vi "一体站流程自动启动.vi"(11 "参数":T1) -> ()   [LabVIEW 2016, in "PLC.lvlib"]
uses:
  PLC.lvlib
panel:
  out "s? t:f":enum16{"初始化", "采配水启动", "仪器操作", "反冲洗", "结束"}(ring)
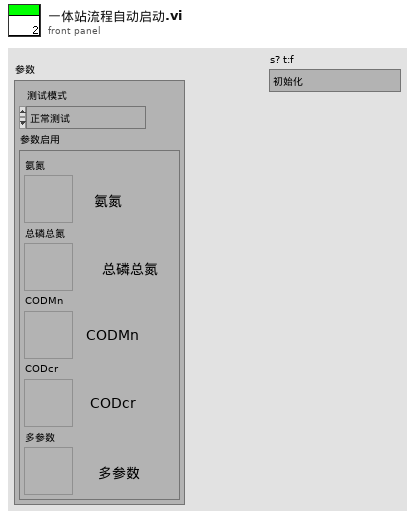
[diagram p1: front panel]
types:
  T1 = cluster{"测试模式":enum16{"正常测试", "集成干预"}, "参数启用":cluster{"氨氮":bool, "总磷总氮":bool, "CODMn":bool, "CODcr":bool, "多参数":bool}}
  T2 = cluster{"命令":string, cluster{"starting address":u16, "holding register value":u16}}
  T3 = enum16{"启动测量", "标样核查", "零点核查", "跨度核查", "空白测试", "平行样测试", "加标回收", "空白校准", "标样校准", "初始化（清洗）", "停止测试", "仪器重启", "校时", "模式设置", "测量间隔设置"}
  T4 = cluster{"站号":u16, "量程切换":enum32{"H", "L", "AUTO"}, "控制命令":enum16{"启动测量", "标样核查", "零点核查", "跨度核查", "空白测试", "平行样测试", "加标回收", "空白校准", "标样校准", "初始化（清洗）", "停止测试", "仪器重启", "校时", "模式设置", "测量间隔设置"}, "模式设置":enum16{"待机", "连续模式", "周期模式", "定点模式", "受控模式", "手动模式"}, "测量间隔":u16}
  T5 = cluster{"时间标识":timestamp, "设备":string, "日志信息":string, "流程参数":string}
  T6 = cluster{"测量模式":enum16{"水样测量", "标样核查", "零点核查", "跨度核查", "空白测试", "加标回收", "平行样", "校零", "校标"}}
  T7 = cluster{"时间标识":timestamp, "设备":string, "日志信息":string}
  T8 = enum16{"空闲", "水样测试", "标样核查", "零点核查", "跨度核查", "空白测试", "平行样测试", "加标回收", "空白校准", "标样校准", "初始化（清洗）"}
  T9 = cluster{"R0":i16, "R1":i16, "R2":i16, "R3":i16, "R4":i16, "R5":i16, "R6":i16, "R7":i16, "R8":i16, "R9":i16, "R10":i16, "R11":i16, "R12":i16, "R13":i16, "R14":i16, "R15":i16, "R16":i16, "R17":i16, "R18":i16, "R19":i16, "R20":i16, "R21":i16, "R22":i16, "R23":i16, "R24":i16, "R25":i16, "R26":i16, "R27":i16, "R28":i16, "R29":i16, "R30":i16, "R31":i16, "R32":i16, "R33":i16, "R34":i16}
  T10 = enum32{"Bad", "Idle", "Run top level", "Running"}
  T11 = cluster{"水样测试量程模式":enum16{"H", "L", "AUTO"}, "空白核查量程模式":enum16{"H", "L", "AUTO"}, "跨度核查量程模式":enum16{"H", "L", "AUTO"}}
  T12 = cluster{"氨氮":bool, "总磷总氮":bool, "CODMn":bool, "CODcr":bool, "多参数":bool}
  T13 = cluster{"水温":dbl, "pH":dbl, "DO":dbl, "Cond":dbl, "Turb":dbl, "叶绿素":dbl, "藻密度":dbl, "蓝绿藻":dbl, "ORP":dbl, "NH3N":dbl}
  T14 = cluster{"时间标识":timestamp, "参数":string, "集成干预测试浓度值":dbl, "集成干预前测试时间":timestamp, "集成干预前测试浓度值":dbl}
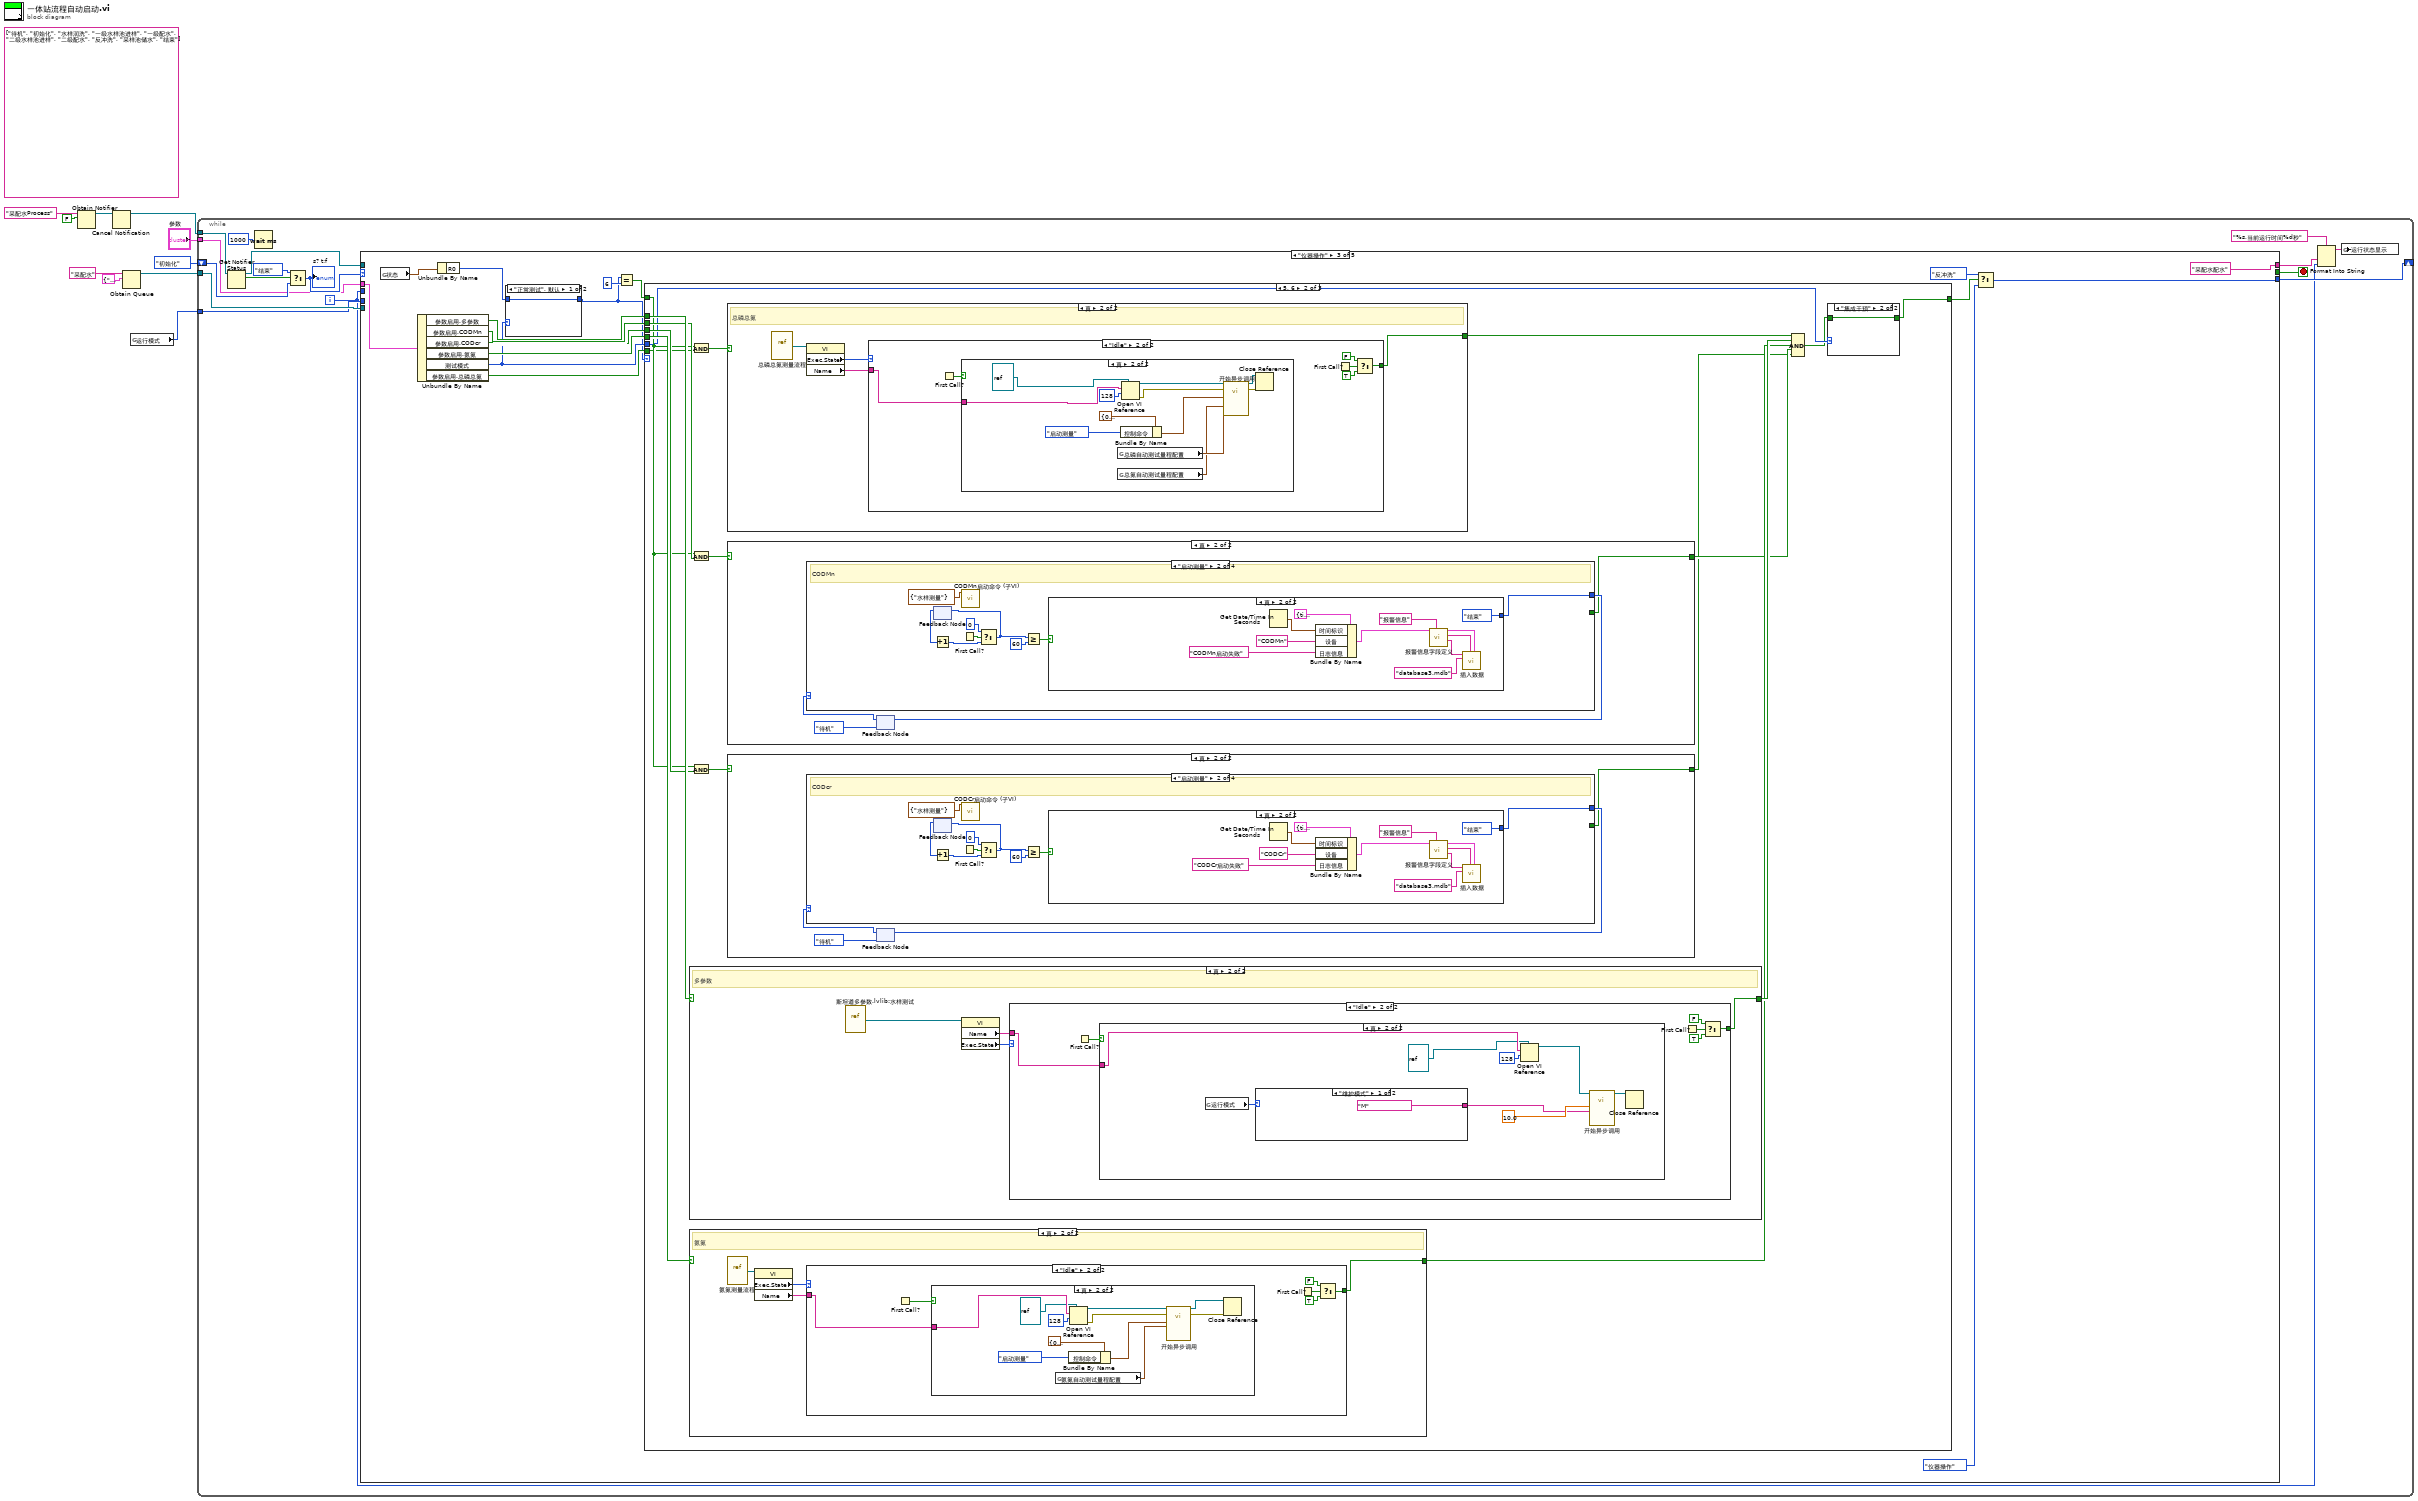
[diagram p0: block diagram]
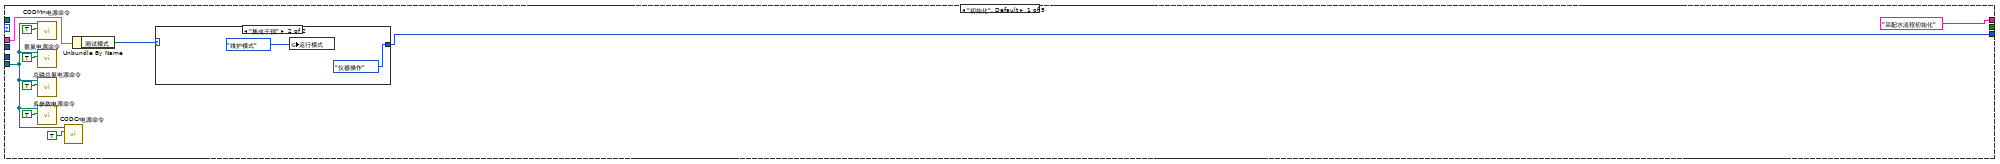
[diagram p2: hidden frame]
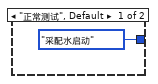
[diagram p3: hidden frame]
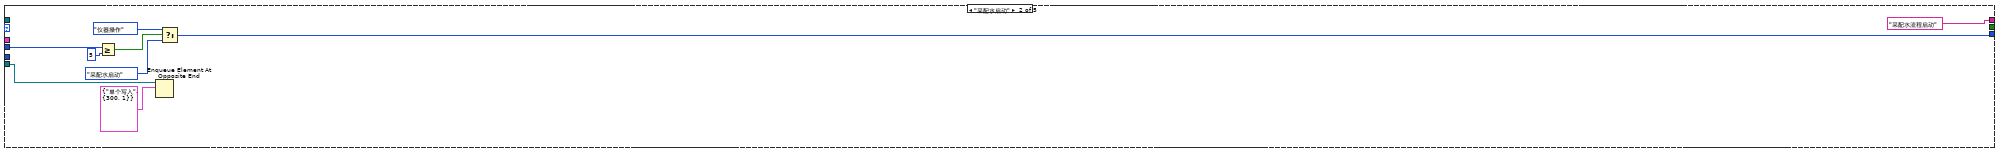
[diagram p4: hidden frame]
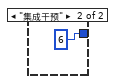
[diagram p5: hidden frame]
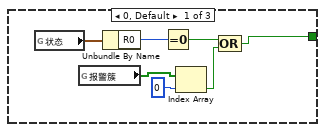
[diagram p6: hidden frame]
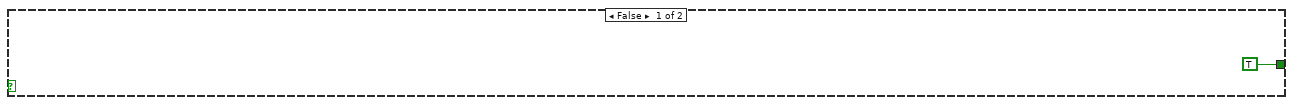
[diagram p7: hidden frame]
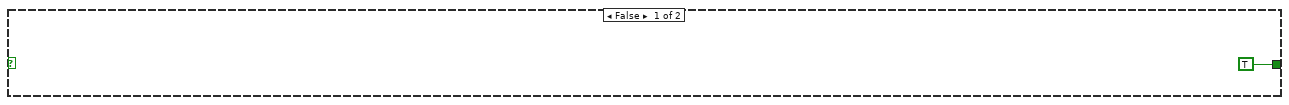
[diagram p11: hidden frame]
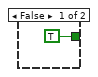
[diagram p14: hidden frame]
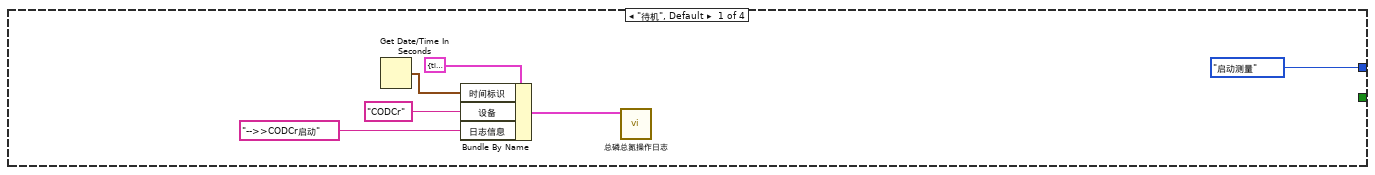
[diagram p15: hidden frame]
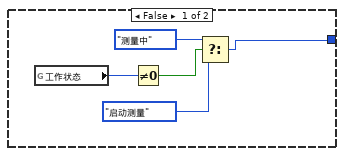
[diagram p16: hidden frame]
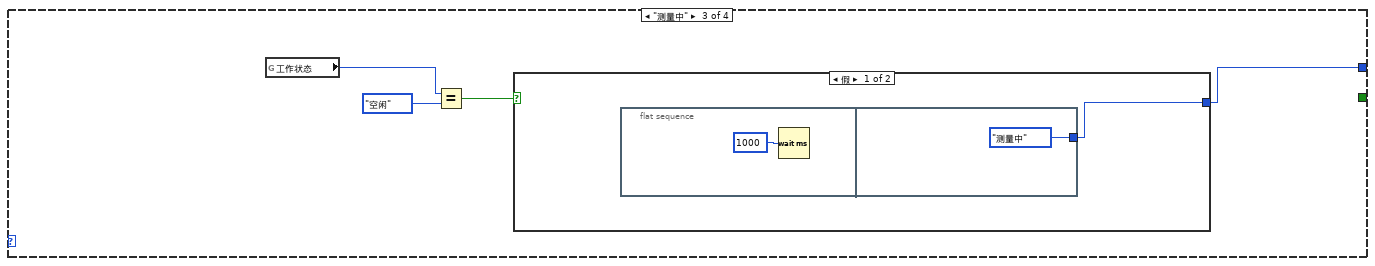
[diagram p17: hidden frame]
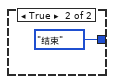
[diagram p18: hidden frame]
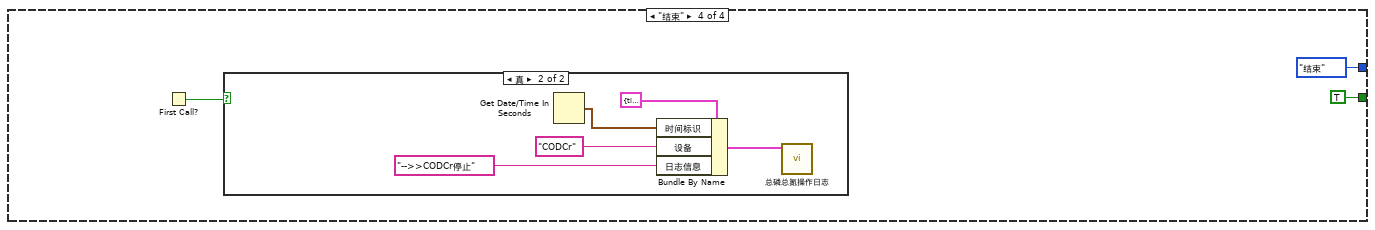
[diagram p19: hidden frame]
diagram:
  (unwired) string[][] [["待机"], ["初始化"], ["水样润洗"], ["一级水样池进样"], ["一级配水"], ["二级水样池进样"], ["二级配水"], ["反冲洗"], ["采样池储水"], ["结束"]] ("项名")
  n1 = Obtain Notifier(name (unnamed)="采配水Process" ("名称（未命名）"), notification data type=FALSE) -> (notifier out=w4:refnum<notifier>)  [unwired: 2 in, 2 out]
  n2 = Cancel Notification(0:w4) -> (8:w3:refnum<notifier>)  [unwired: 1 in, 2 out]
  n3 = Obtain Queue(name (unnamed)="采配水" ("名称（未命名）"), element data type=cluster{"命令":string, "数据":variant} {"命令"="", "数据"=variant}) -> (queue out=w7:refnum<queue>)  [unwired: 3 in, 2 out]
  n4 = global read "系统设置全局变量.vi" "运行模式"() -> (w1:enum16{"维护模式", "常规模式", "应急模式", "质控模式"})
  n5 = while {
    shift-right: [w23] -> _
    shift-left: enum16{"初始化", "采配水启动", "仪器操作", "反冲洗", "结束"}."初始化" ("枚举") -> [w19]
    tunnel: w7 -> [w26]
    tunnel: w3 -> [w22]
    tunnel: "参数" -> [w13]
    tunnel: w1 -> [w12]
    i -> [w11]
    stop <- w25 stop-if-true
    n6 = Get Notifier Status(notifier=w22) -> (notifier out=w14:refnum<notifier>, current notification=w21:bool)  [unwired: 1 in, 3 out]
    n7 = Wait (ms)(milliseconds to wait=u32 1000 ("等待时间（毫秒）")) -> ()  [unwired: 1 out]
    n8 = Select(t=enum16{"初始化", "采配水启动", "仪器操作", "反冲洗", "结束"}."结束" ("枚举"), s=w21, f=w19) -> (s? t:f=w18:enum16{"初始化", "采配水启动", "仪器操作", "反冲洗", "结束"})
    "s? t:f" <- w18
    n9 = case shown="\"仪器操作\"" w18 {
      tunnel: w26 -> [w31 w48 _ _ w442]
      tunnel: [_ _ _ _ TRUE] -> w25
      tunnel: [w30 w40 w60 w266 enum16{"初始化", "采配水启动", "仪器操作", "反冲洗", "结束"}."结束" ("枚举")] -> w23
      tunnel: ["采配水流程初始化" "采配水流程启动" "采配水配水" "等待测试完成" "采配水结束"] -> w15
      tunnel: w14 -> [_ _ _ _ w443]
      tunnel: w13 -> [w28 _ w63 w265 w439]
      tunnel: w12 -> [_ _ _ _ w438]
      tunnel: w11 -> [_ w46 _ _ _]
      frame "初始化", Default {
        n10 = call "CODMn电源命令.vi"("通电/断电"=TRUE, "队列"=w31) -> ()  [unwired: 9 in, 1 out]
        n11 = call "氨氮电源命令.vi"("通电/断电"=TRUE, "队列"=w31) -> ()  [unwired: 9 in, 1 out]
        n12 = call "总磷总氮电源命令.vi"("通电/断电"=TRUE, "队列"=w31) -> ()  [unwired: 9 in, 1 out]
        n13 = call "多参数电源命令.vi"("通电/断电"=TRUE, "队列"=w31) -> ()  [unwired: 9 in, 1 out]
        n14 = call "CODCr电源命令.vi"("通电/断电"=TRUE, "队列"=w31) -> ()  [unwired: 9 in, 1 out]
        n15 = Unbundle By Name(w28) -> ("测试模式"=w27:enum16{"正常测试", "集成干预"})
        n16 = case shown="\"集成干预\"" w27 {
          tunnel: [enum16{"初始化", "采配水启动", "仪器操作", "反冲洗", "结束"}."采配水启动" ("枚举") enum16{"初始化", "采配水启动", "仪器操作", "反冲洗", "结束"}."仪器操作" ("枚举")] -> w30
          frame "正常测试", Default {
          }
          frame "集成干预" {
            n17 = global write "系统设置全局变量.vi" "运行模式"(enum16{"维护模式", "常规模式", "应急模式", "质控模式"}."维护模式" ("运行模式")) -> ()
          }
        }
      }
      frame "采配水启动" {
        n18 = Greater Or Equal?(x=w46, y=5) -> (x >= y?=w43:bool)
        n19 = Enqueue Element At Opposite End(queue=w48, element=T2 {"命令"="单个写入", {"starting address"=300, "holding register value"=1}} ("元素")) -> ()  [unwired: 2 in, 3 out]
        n20 = Select(t=enum16{"初始化", "采配水启动", "仪器操作", "反冲洗", "结束"}."仪器操作" ("枚举"), s=w43, f=enum16{"初始化", "采配水启动", "仪器操作", "反冲洗", "结束"}."采配水启动" ("枚举")) -> (s? t:f=w40:enum16{"初始化", "采配水启动", "仪器操作", "反冲洗", "结束"})
      }
      frame "仪器操作" {
        n21 = global read "采配水全局变量.vi" "状态"() -> (w65:T9)
        n22 = Unbundle By Name(w63) -> ("参数启用.多参数"=w58:bool, "参数启用.CODMn"=w57:bool, "参数启用.CODcr"=w56:bool, "参数启用.氨氮"=w55:bool, "测试模式"=w53:enum16{"正常测试", "集成干预"}, "参数启用.总磷总氮"=w52:bool)
        n23 = Unbundle By Name(w65) -> ("R0"=w54:i16)
        n24 = case shown="\"正常测试\", 默认" w53 {
          tunnel: w54 -> [w66 _]
          tunnel: [w66 i16 6 ("R0")] -> w50
          frame "正常测试", Default {
          }
          frame "集成干预" {
          }
        }
        n25 = Equal?(x=w50, y=i16 6) -> (x = y?=w49:bool)
        n26 = case shown="5, 6" w50 {
          tunnel: [w69 w79 TRUE] -> w62
          tunnel: w58 -> [_ w91 _]
          tunnel: w57 -> [_ w90 _]
          tunnel: w56 -> [_ w87 _]
          tunnel: w55 -> [_ w86 _]
          tunnel: w49 -> [_ w78 _]
          tunnel: w53 -> [_ w81 _]
          tunnel: w52 -> [_ w77 _]
          frame 0, Default {
            n27 = global read "采配水全局变量.vi" "状态"() -> (w72:T9)
            n28 = global read "采配水全局变量.vi" "报警簇"() -> (w73:bool[])
            n29 = Unbundle By Name(w72) -> ("R0"=w71:i16)
            n30 = Equal To 0?(x=w71) -> (x = 0?=w74:bool)
            n31 = Index Array(array=w73, index=0 ("索引")) -> (element=w68:bool)
            n32 = Compound Arithmetic op=OR ("复合运算")(w74, w68) -> (w69:bool)
          }
          frame 5, 6 {
            n33 = case shown="真" w91 {
              tunnel: [TRUE ("t") w242] -> w85
              frame False {
              }
              frame True {
                # "多参数"
                n34 = vi-ref "斯坦道多参数.lvlib:水样测试.vi"() -> (w244:refnum<vi>)
                n35 = property class="VI"(reference=w244) -> ("Name"=w243:string, "Exec.State"=w245:T10)  [unwired: 1 in, 2 out]
                n36 = case shown="\"Idle\"" w245 {
                  tunnel: w243 -> [_ w251]
                  tunnel: [_ w246] -> w242
                  frame "Bad", Default {
                  }
                  frame "Idle" {
                    n37 = First Call?() -> (First Call?: T/F=w250:bool)
                    n38 = case shown="真" w250 {
                      tunnel: w251 -> [_ w258]
                      frame False {
                      }
                      frame True {
                        n39 = global read "系统设置全局变量.vi" "运行模式"() -> (w255:enum16{"维护模式", "常规模式", "应急模式", "质控模式"})
                        n40 = case shown="\"维护模式\"" w255 {
                          tunnel: ["M" ("数据标记表") "N" ("数据标记表")] -> w252
                          frame "维护模式" {
                          }
                          frame "常规模式", Default {
                          }
                        }
                        n41 = Open VI Reference(type specifier VI Refnum (for type only)=refnum<vi> refnum, vi path=w258, options=128 ("选项")) -> (vi reference=w257:refnum<vi>)  [unwired: 3 in, 1 out]
                        n42 = call-by-ref "开始异步调用"(reference=w257, "数据标记表"=w252, "水样测试时间"=10.0 ("测量时间")) -> (reference out=w256:refnum<vi>)  [unwired: 11 in, 1 out]
                        n43 = Close Reference(reference=w256) -> ()  [unwired: 1 in, 1 out]
                      }
                    }
                    n44 = First Call?() -> (First Call?: T/F=w249:bool)
                    n45 = Select(t=FALSE, s=w249, f=TRUE) -> (s? t:f=w246:bool)
                  }
                }
              }
            }
            n46 = case "条件结构" shown="真" w86 {
              tunnel: [TRUE ("t") w117] -> w84
              frame False {
              }
              frame True {
                # "氨氮"
                n47 = vi-ref "氨氮测量流程.vi"() -> (w120:refnum<vi>)
                n48 = property class="VI"(reference=w120) -> ("Exec.State"=w119:T10, "Name"=w118:string)  [unwired: 1 in, 2 out]
                n49 = case shown="\"Idle\"" w119 {
                  tunnel: w118 -> [_ w126]
                  tunnel: [_ w121] -> w117
                  frame "Bad", Default {
                  }
                  frame "Idle" {
                    n50 = First Call?() -> (First Call?: T/F=w125:bool)
                    n51 = case shown="真" w125 {
                      tunnel: w126 -> [_ w134]
                      frame False {
                      }
                      frame True {
                        n52 = global read "氨氮断电保存全局变量.vi" "氨氮自动测试量程配置"() -> (w127:T11)
                        n53 = Bundle By Name(cluster=T4 {"站号"=0, "量程切换"=enum."H", "控制命令"=enum."启动测量", "模式设置"=enum."待机", "测量间隔"=0} ("参数"), "控制命令"=T3."启动测量") -> (w129:T4)
                        n54 = Open VI Reference(type specifier VI Refnum (for type only)=refnum<vi> refnum, vi path=w134, options=128 ("选项")) -> (vi reference=w130:refnum<vi>, error out=w135:errorcluster)  [unwired: 3 in]
                        n55 = call-by-ref "开始异步调用"(reference=w130, error in=w135, "量程模式"=w127, "参数"=w129) -> (reference out=w136:refnum<vi>, error out=w137:errorcluster)  [unwired: 10 in]
                        n56 = Close Reference(reference=w136, error in (no error)=w137) -> ()  [unwired: 1 out]
                      }
                    }
                    n57 = First Call?() -> (First Call?: T/F=w124:bool)
                    n58 = Select(t=FALSE, s=w124, f=TRUE) -> (s? t:f=w121:bool)
                  }
                }
              }
            }
            n59 = And(x=w78, y=w77) -> (x .and. y?=w76:bool)
            n60 = And(x=w78, y=w90) -> (x .and. y?=w89:bool)
            n61 = And(x=w78, y=w87) -> (x .and. y?=w88:bool)
            n62 = case "条件结构" shown="真" w76 {
              tunnel: [TRUE ("t") w93] -> w75
              frame False {
              }
              frame True {
                # "总磷总氮"
                n63 = vi-ref "总磷总氮测量流程.vi"() -> (w96:refnum<vi>)
                n64 = property class="VI"(reference=w96) -> ("Exec.State"=w95:T10, "Name"=w94:string)  [unwired: 1 in, 2 out]
                n65 = case shown="\"Idle\"" w95 {
                  tunnel: w94 -> [_ w102]
                  tunnel: [_ w97] -> w93
                  frame "Bad", Default {
                  }
                  frame "Idle" {
                    n66 = First Call?() -> (First Call?: T/F=w101:bool)
                    n67 = case shown="真" w101 {
                      tunnel: w102 -> [_ w111]
                      frame False {
                      }
                      frame True {
                        n68 = global read "总磷总氮断电保存全局变量.vi" "总磷自动测试量程配置"() -> (w105:T11)
                        n69 = global read "总磷总氮断电保存全局变量.vi" "总氮自动测试量程配置"() -> (w104:T11)
                        n70 = Bundle By Name(cluster=T4 {"站号"=0, "量程切换"=enum."H", "控制命令"=enum."启动测量", "模式设置"=enum."待机", "测量间隔"=0} ("参数"), "控制命令"=T3."启动测量") -> (w106:T4)
                        n71 = Open VI Reference(type specifier VI Refnum (for type only)=refnum<vi> refnum, vi path=w111, options=128 ("选项")) -> (vi reference=w107:refnum<vi>, error out=w112:errorcluster)  [unwired: 3 in]
                        n72 = call-by-ref "开始异步调用"(reference=w107, error in=w112, "总氮量程模式"=w104, "总磷量程模式"=w105, "参数"=w106) -> (reference out=w113:refnum<vi>, error out=w114:errorcluster)  [unwired: 9 in]
                        n73 = Close Reference(reference=w113, error in (no error)=w114) -> ()  [unwired: 1 out]
                      }
                    }
                    n74 = First Call?() -> (First Call?: T/F=w100:bool)
                    n75 = Select(t=FALSE, s=w100, f=TRUE) -> (s? t:f=w97:bool)
                  }
                }
              }
            }
            n76 = case shown="真" w89 {
              tunnel: [TRUE w191] -> w83
              frame False {
              }
              frame True {
                n77 = feedback #1(enum16{"待机", "启动测量", "测量中", "结束"}."待机") -> (w193:enum16{"待机", "启动测量", "测量中", "结束"})
                n78 = case shown="\"启动测量\"" w193 {
                  tunnel: [enum16{"待机", "启动测量", "测量中", "结束"}."启动测量" w209 w228 enum16{"待机", "启动测量", "测量中", "结束"}."结束"] -> w192
                  tunnel: [_ _ _ TRUE] -> w191
                  frame "待机", Default {
                    n79 = Get Date/Time In Seconds() -> (seconds since 1Jan1904=w199:timestamp)
                    n80 = Bundle By Name(cluster=T5 {"时间标识"=timestamp(0 s since 1904-01-01), "设备"="", "日志信息"="", "流程参数"=""} ("data in"), "时间标识"=w199, "设备"="CODMn", "日志信息"="-->>CODMn启动") -> (w195:T5)
                    n81 = call "总磷总氮操作日志.vi"("data in"=w195) -> ()  [unwired: 11 in]
                  }
                  frame "启动测量" {
                    # "CODMn"
                    n82 = feedback #2() -> (w205:i32)  [unwired: 1 in]
                    n83 = Increment(x=w205) -> (x+1=w206:i32)
                    n84 = First Call?() -> (First Call?: T/F=w204:bool)
                    n85 = call "CODMn启动命令 (子VI).vi"("启动测量模式"=T6 {"测量模式"=enum."水样测量"}) -> ()  [unwired: 11 in]
                    n86 = Select(t=0, s=w204, f=w206) -> (s? t:f=w207:i32)
                    n87 = feedback-in #2(w207) -> ()
                    n88 = Greater Or Equal?(x=w207, y=60) -> (x >= y?=w202:bool)
                    n89 = case shown="真" w202 {
                      tunnel: [w211 enum16{"待机", "启动测量", "测量中", "结束"}."结束"] -> w209
                      frame False {
                        n90 = global read "运行时序全局变量.vi" "多列列表框"() -> (w210:i32)
                        n91 = Not Equal To 0?(x=w210) -> (x != 0?=w212:bool)
                        n92 = Select(t=enum16{"待机", "启动测量", "测量中", "结束"}."测量中", s=w212, f=enum16{"待机", "启动测量", "测量中", "结束"}."启动测量") -> (s? t:f=w211:enum16{"待机", "启动测量", "测量中", "结束"})
                      }
                      frame True {
                        n93 = Get Date/Time In Seconds() -> (seconds since 1Jan1904=w221:timestamp)
                        n94 = Bundle By Name(cluster=T7 {"时间标识"=timestamp(0 s since 1904-01-01), "设备"="", "日志信息"=""} ("data in"), "时间标识"=w221, "设备"="CODMn", "日志信息"="CODMn启动失败") -> (w215:T7)
                        n95 = call "报警信息字段定义.vi"("table输入"="报警信息", "data in"=w215) -> ("table输出"=w218:string, "columns"=w219:string[], "data out"=w220:T7)  [unwired: 7 in]
                        n96 = call "插入数据.vi"("data"=w220, "columns"=w219, "database"="database3.mdb", "table"=w218) -> ()  [unwired: 7 in, 1 out]
                      }
                    }
                  }
                  frame "测量中" {
                    n97 = global read "运行时序全局变量.vi" "多列列表框"() -> (w227:i32)
                    n98 = Equal To 0?(x=w227) -> (x = 0?=w226:bool)
                    n99 = case shown="假" w226 {
                      tunnel: [w229 enum16{"待机", "启动测量", "测量中", "结束"}."结束"] -> w228
                      frame False {
                        n100 = flat-sequence {
                          tunnel: [enum16{"待机", "启动测量", "测量中", "结束"}."测量中"] -> w229
                          frame #0 {
                            n101 = Wait (ms)(milliseconds to wait=u32 1000 ("等待时间（毫秒）")) -> ()  [unwired: 1 out]
                          }
                          frame #1 {
                          }
                        }
                      }
                      frame True {
                      }
                    }
                  }
                  frame "结束" {
                    n102 = First Call?() -> (First Call?: T/F=w233:bool)
                    n103 = case shown="真" w233 {
                      frame False {
                      }
                      frame True {
                        n104 = Get Date/Time In Seconds() -> (seconds since 1Jan1904=w240:timestamp)
                        n105 = Bundle By Name(cluster=T5 {"时间标识"=timestamp(0 s since 1904-01-01), "设备"="", "日志信息"="", "流程参数"=""} ("data in"), "时间标识"=w240, "设备"="CODMn", "日志信息"="-->>CODMn停止") -> (w236:T5)
                        n106 = call "总磷总氮操作日志.vi"("data in"=w236) -> ()  [unwired: 11 in]
                      }
                    }
                  }
                }
                n107 = feedback-in #1(w192) -> ()
              }
            }
            n108 = case shown="真" w88 {
              tunnel: [TRUE w139] -> w82
              frame False {
              }
              frame True {
                n109 = feedback #3(enum16{"待机", "启动测量", "测量中", "结束"}."待机") -> (w141:enum16{"待机", "启动测量", "测量中", "结束"})
                n110 = case shown="\"启动测量\"" w141 {
                  tunnel: [enum16{"待机", "启动测量", "测量中", "结束"}."启动测量" w157 w177 enum16{"待机", "启动测量", "测量中", "结束"}."结束"] -> w140
                  tunnel: [_ _ _ TRUE] -> w139
                  frame "待机", Default {
                    n111 = Get Date/Time In Seconds() -> (seconds since 1Jan1904=w147:timestamp)
                    n112 = Bundle By Name(cluster=T5 {"时间标识"=timestamp(0 s since 1904-01-01), "设备"="", "日志信息"="", "流程参数"=""} ("data in"), "时间标识"=w147, "设备"="CODCr", "日志信息"="-->>CODCr启动") -> (w143:T5)
                    n113 = call "总磷总氮操作日志.vi"("data in"=w143) -> ()  [unwired: 11 in]
                  }
                  frame "启动测量" {
                    # "CODcr"
                    n114 = feedback #4() -> (w153:i32)  [unwired: 1 in]
                    n115 = Increment(x=w153) -> (x+1=w154:i32)
                    n116 = First Call?() -> (First Call?: T/F=w152:bool)
                    n117 = call "CODCr启动命令 (子VI).vi"("启动测量模式"=T6 {"测量模式"=enum."水样测量"}) -> ()  [unwired: 11 in]
                    n118 = Select(t=0, s=w152, f=w154) -> (s? t:f=w155:i32)
                    n119 = feedback-in #4(w155) -> ()
                    n120 = Greater Or Equal?(x=w155, y=60) -> (x >= y?=w150:bool)
                    n121 = case shown="真" w150 {
                      tunnel: [w158 enum16{"待机", "启动测量", "测量中", "结束"}."结束"] -> w157
                      frame False {
                        n122 = global read "CODcr全局变量.vi" "工作状态"() -> (w159:T8)
                        n123 = Not Equal To 0?(x=w159) -> (x != 0?=w160:bool)
                        n124 = Select(t=enum16{"待机", "启动测量", "测量中", "结束"}."测量中", s=w160, f=enum16{"待机", "启动测量", "测量中", "结束"}."启动测量") -> (s? t:f=w158:enum16{"待机", "启动测量", "测量中", "结束"})
                      }
                      frame True {
                        n125 = Get Date/Time In Seconds() -> (seconds since 1Jan1904=w169:timestamp)
                        n126 = Bundle By Name(cluster=T7 {"时间标识"=timestamp(0 s since 1904-01-01), "设备"="", "日志信息"=""} ("data in"), "时间标识"=w169, "设备"="CODCr", "日志信息"="CODCr启动失败") -> (w163:T7)
                        n127 = call "报警信息字段定义.vi"("table输入"="报警信息", "data in"=w163) -> ("table输出"=w166:string, "columns"=w167:string[], "data out"=w168:T7)  [unwired: 7 in]
                        n128 = call "插入数据.vi"("data"=w168, "columns"=w167, "database"="database3.mdb", "table"=w166) -> ()  [unwired: 7 in, 1 out]
                      }
                    }
                  }
                  frame "测量中" {
                    n129 = global read "CODcr全局变量.vi" "工作状态"() -> (w176:T8)
                    n130 = Equal?(x=w176, y=T8."空闲" ("工作状态")) -> (x = y?=w175:bool)
                    n131 = case shown="假" w175 {
                      tunnel: [w178 enum16{"待机", "启动测量", "测量中", "结束"}."结束"] -> w177
                      frame False {
                        n132 = flat-sequence {
                          tunnel: [enum16{"待机", "启动测量", "测量中", "结束"}."测量中"] -> w178
                          frame #0 {
                            n133 = Wait (ms)(milliseconds to wait=u32 1000 ("等待时间（毫秒）")) -> ()  [unwired: 1 out]
                          }
                          frame #1 {
                          }
                        }
                      }
                      frame True {
                      }
                    }
                  }
                  frame "结束" {
                    n134 = First Call?() -> (First Call?: T/F=w182:bool)
                    n135 = case shown="真" w182 {
                      frame False {
                      }
                      frame True {
                        n136 = Get Date/Time In Seconds() -> (seconds since 1Jan1904=w189:timestamp)
                        n137 = Bundle By Name(cluster=T5 {"时间标识"=timestamp(0 s since 1904-01-01), "设备"="", "日志信息"="", "流程参数"=""} ("data in"), "时间标识"=w189, "设备"="CODCr", "日志信息"="-->>CODCr停止") -> (w185:T5)
                        n138 = call "总磷总氮操作日志.vi"("data in"=w185) -> ()  [unwired: 11 in]
                      }
                    }
                  }
                }
                n139 = feedback-in #3(w140) -> ()
              }
            }
            n140 = Compound Arithmetic op=AND ("复合运算")(w75, w85, w84, w83, w82) -> (w80:bool)
            n141 = case shown="\"集成干预\"" w81 {
              tunnel: w80 -> [_ w115]
              tunnel: [_ w115] -> w79
              frame "正常测试", Default {
              }
              frame "集成干预" {
              }
            }
          }
          frame 7..9 {
          }
        }
        n142 = Select(t=enum16{"初始化", "采配水启动", "仪器操作", "反冲洗", "结束"}."反冲洗" ("枚举"), s=w62, f=enum16{"初始化", "采配水启动", "仪器操作", "反冲洗", "结束"}."仪器操作" ("枚举")) -> (s? t:f=w60:enum16{"初始化", "采配水启动", "仪器操作", "反冲洗", "结束"})
      }
      frame "反冲洗" {
        n143 = First Call?() -> (First Call?: T/F=w263:bool)
        n144 = case shown="真" w263 {
          tunnel: w265 -> [_ w274]
          frame False {
          }
          frame True {
            n145 = Unbundle By Name(w274) -> ("测试模式"=w273:enum16{"正常测试", "集成干预"}, "参数启用"=w272:T12)
            n146 = case shown="\"正常测试\", 默认" w273 {
              tunnel: w272 -> [w277 w369]
              frame "正常测试", Default {
                n147 = global read "系统设置全局变量.vi" "运行模式"() -> (w275:enum16{"维护模式", "常规模式", "应急模式", "质控模式"})
                n148 = global read "采配水全局变量.vi" "报警簇"() -> (w282:bool[])
                n149 = case shown="\"维护模式\"" w275 {
                  tunnel: ["M" ("table") "N" ("table")] -> w276
                  frame "维护模式" {
                  }
                  frame "常规模式", Default {
                  }
                }
                n150 = Index Array(array=w282, index #1=0 ("索引"), index #2=11 ("索引")) -> (element #1=w279:bool, element #2=w278:bool)
                n151 = case shown="真" w279 {
                  tunnel: w278 -> [w288 _]
                  tunnel: w277 -> [w287 w301]
                  tunnel: w276 -> [w285 w295]
                  frame False {
                    n152 = Unbundle By Name(w287) -> ("氨氮"=w286:bool)
                    n153 = case shown="真" w288 {
                      tunnel: w286 -> [_ w290]
                      tunnel: w285 -> [_ w289]
                      frame False {
                      }
                      frame True {
                        n154 = case shown="真" w290 {
                          tunnel: w289 -> [_ w291]
                          tunnel: [_ w292] -> _
                          frame False {
                          }
                          frame True {
                            n155 = call "取水点无水样数据存储.vi"("数据标识"="lw", "数据类型"=w291, "table"="氨氮") -> ("error out"=w292:errorcluster)  [unwired: 8 in]
                          }
                        }
                      }
                    }
                  }
                  frame True {
                    n156 = Unbundle By Name(w301) -> ("氨氮"=w300:bool, "CODMn"=w299:bool, "CODcr"=w298:bool, "多参数"=w297:bool, "总磷总氮"=w296:bool)
                    n157 = case shown="真" w300 {
                      tunnel: w295 -> [_ w361]
                      tunnel: [_ w362] -> _
                      frame False {
                      }
                      frame True {
                        n158 = call "取水点无水样数据存储.vi"("数据标识"="Z", "数据类型"=w361, "table"="氨氮") -> ("error out"=w362:errorcluster)  [unwired: 8 in]
                      }
                    }
                    n159 = case shown="真" w299 {
                      tunnel: w295 -> [_ w358]
                      tunnel: [_ w357] -> _
                      frame False {
                      }
                      frame True {
                        n160 = call "取水点无水样数据存储.vi"("数据标识"="Z", "数据类型"=w358, "table"="CODMn") -> ("error out"=w357:errorcluster)  [unwired: 8 in]
                      }
                    }
                    n161 = case shown="真" w298 {
                      tunnel: w295 -> [_ w354]
                      tunnel: [_ w353] -> _
                      frame False {
                      }
                      frame True {
                        n162 = call "取水点无水样数据存储.vi"("数据标识"="Z", "数据类型"=w354, "table"="CODCr") -> ("error out"=w353:errorcluster)  [unwired: 8 in]
                      }
                    }
                    n163 = case shown="真" w296 {
                      tunnel: w295 -> [_ w303]
                      tunnel: [_ w302] -> _
                      frame False {
                      }
                      frame True {
                        n164 = call "取水点无水样数据存储.vi"("数据标识"="Z", "数据类型"=w303, "table"="总氮") -> ("error out"=w304:errorcluster)  [unwired: 8 in]
                        n165 = call "取水点无水样数据存储.vi"("error in (no error)"=w304, "数据标识"="Z", "数据类型"=w303, "table"="总磷") -> ("error out"=w302:errorcluster)  [unwired: 7 in]
                      }
                    }
                    n166 = case shown="真" w297 {
                      tunnel: w295 -> [_ w309]
                      frame False {
                      }
                      frame True {
                        n167 = global read "多参数全局变量.vi" "传感器通道号"() -> (w324:T13)
                        n168 = Unbundle By Name(w324) -> ("水温"=w323:dbl, "pH"=w322:dbl, "DO"=w321:dbl, "Cond"=w320:dbl, "Turb"=w319:dbl, "叶绿素"=w318:dbl, "藻密度"=w317:dbl)
                        n169 = Not Equal To 0?(x=w323) -> (x != 0?=w316:bool)
                        n170 = Not Equal To 0?(x=w322) -> (x != 0?=w315:bool)
                        n171 = Not Equal To 0?(x=w321) -> (x != 0?=w314:bool)
                        n172 = Not Equal To 0?(x=w320) -> (x != 0?=w313:bool)
                        n173 = Not Equal To 0?(x=w319) -> (x != 0?=w312:bool)
                        n174 = Not Equal To 0?(x=w318) -> (x != 0?=w311:bool)
                        n175 = Not Equal To 0?(x=w317) -> (x != 0?=w310:bool)
                        n176 = case shown="真" w316 {
                          tunnel: w309 -> [_ w350]
                          tunnel: [_ w349] -> _
                          frame False {
                          }
                          frame True {
                            n177 = call "取水点无水样数据存储.vi"("数据标识"="Z", "数据类型"=w350, "table"="水温") -> ("error out"=w349:errorcluster)  [unwired: 8 in]
                          }
                        }
                        n178 = case shown="真" w315 {
                          tunnel: w309 -> [_ w346]
                          tunnel: [_ w345] -> _
                          frame False {
                          }
                          frame True {
                            n179 = call "取水点无水样数据存储.vi"("数据标识"="Z", "数据类型"=w346, "table"="pH") -> ("error out"=w345:errorcluster)  [unwired: 8 in]
                          }
                        }
                        n180 = case shown="真" w314 {
                          tunnel: w309 -> [_ w342]
                          tunnel: [_ w341] -> _
                          frame False {
                          }
                          frame True {
                            n181 = call "取水点无水样数据存储.vi"("数据标识"="Z", "数据类型"=w342, "table"="DO") -> ("error out"=w341:errorcluster)  [unwired: 8 in]
                          }
                        }
                        n182 = case shown="真" w312 {
                          tunnel: w309 -> [_ w334]
                          tunnel: [_ w333] -> _
                          frame False {
                          }
                          frame True {
                            n183 = call "取水点无水样数据存储.vi"("数据标识"="Z", "数据类型"=w334, "table"="浊度") -> ("error out"=w333:errorcluster)  [unwired: 8 in]
                          }
                        }
                        n184 = case shown="真" w313 {
                          tunnel: w309 -> [_ w338]
                          tunnel: [_ w337] -> _
                          frame False {
                          }
                          frame True {
                            n185 = call "取水点无水样数据存储.vi"("数据标识"="Z", "数据类型"=w338, "table"="比电导率") -> ("error out"=w337:errorcluster)  [unwired: 8 in]
                          }
                        }
                        n186 = case shown="真" w311 {
                          tunnel: w309 -> [_ w330]
                          tunnel: [_ w329] -> _
                          frame False {
                          }
                          frame True {
                            n187 = call "取水点无水样数据存储.vi"("数据标识"="Z", "数据类型"=w330, "table"="叶绿素") -> ("error out"=w329:errorcluster)  [unwired: 8 in]
                          }
                        }
                        n188 = case shown="真" w310 {
                          tunnel: w309 -> [_ w326]
                          tunnel: [_ w325] -> _
                          frame False {
                          }
                          frame True {
                            n189 = call "取水点无水样数据存储.vi"("数据标识"="Z", "数据类型"=w326, "table"="藻密度") -> ("error out"=w325:errorcluster)  [unwired: 8 in]
                          }
                        }
                      }
                    }
                  }
                }
              }
              frame "集成干预" {
                n190 = Unbundle By Name(w369) -> ("氨氮"=w368:bool, "CODMn"=w367:bool, "CODcr"=w366:bool, "多参数"=w365:bool)
                n191 = case shown="真" w368 {
                  frame False {
                  }
                  frame True {
                    n192 = call "获取最近两组水样测试数据.vi"("table"="氨氮") -> ("error out"=w435:errorcluster, "存储变量"=w436:T14)  [unwired: 9 in]
                    n193 = call "集成干预测试数据存储.vi"("error in (no error)"=w435, "存储变量"=w436) -> ("error out"=w431:errorcluster)  [unwired: 9 in]
                    n194 = call "获取最近两组水样测试数据.vi"("error in (no error)"=w431, "table"="总磷") -> ("error out"=w434:errorcluster, "存储变量"=w433:T14)  [unwired: 8 in]
                    n195 = call "集成干预测试数据存储.vi"("error in (no error)"=w434, "存储变量"=w433) -> ()  [unwired: 9 in, 1 out]
                  }
                }
                n196 = case shown="真" w367 {
                  frame False {
                  }
                  frame True {
                    n197 = call "获取最近两组水样测试数据.vi"("table"="CODMn") -> ("error out"=w428:errorcluster, "存储变量"=w429:T14)  [unwired: 9 in]
                    n198 = call "集成干预测试数据存储.vi"("error in (no error)"=w428, "存储变量"=w429) -> ()  [unwired: 9 in, 1 out]
                  }
                }
                n199 = case shown="真" w366 {
                  frame False {
                  }
                  frame True {
                    n200 = call "获取最近两组水样测试数据.vi"("table"="CODCr") -> ("error out"=w425:errorcluster, "存储变量"=w426:T14)  [unwired: 9 in]
                    n201 = call "集成干预测试数据存储.vi"("error in (no error)"=w425, "存储变量"=w426) -> ()  [unwired: 9 in, 1 out]
                  }
                }
                n202 = case shown="真" w365 {
                  frame False {
                  }
                  frame True {
                    n203 = global read "多参数全局变量.vi" "传感器通道号"() -> (w390:T13)
                    n204 = Unbundle By Name(w390) -> ("水温"=w389:dbl, "pH"=w386:dbl, "DO"=w383:dbl, "Cond"=w380:dbl, "Turb"=w378:dbl, "叶绿素"=w377:dbl, "藻密度"=w376:dbl)
                    n205 = Not Equal To 0?(x=w389) -> (x != 0?=w388:bool)
                    n206 = Not Equal To 0?(x=w386) -> (x != 0?=w385:bool)
                    n207 = case shown="真" w388 {
                      tunnel: [_ w421] -> w387
                      frame False {
                      }
                      frame True {
                        n208 = call "获取最近两组水样测试数据.vi"("table"="水温") -> ("error out"=w424:errorcluster, "存储变量"=w423:T14)  [unwired: 9 in]
                        n209 = call "集成干预测试数据存储.vi"("error in (no error)"=w424, "存储变量"=w423) -> ("error out"=w421:errorcluster)  [unwired: 9 in]
                      }
                    }
                    n210 = Not Equal To 0?(x=w376) -> (x != 0?=w370:bool)
                    n211 = Not Equal To 0?(x=w377) -> (x != 0?=w372:bool)
                    n212 = Not Equal To 0?(x=w378) -> (x != 0?=w374:bool)
                    n213 = Not Equal To 0?(x=w380) -> (x != 0?=w379:bool)
                    n214 = Not Equal To 0?(x=w383) -> (x != 0?=w382:bool)
                    n215 = case shown="真" w385 {
                      tunnel: [_ w417] -> w384
                      tunnel: w387 -> [_ w416]
                      frame False {
                      }
                      frame True {
                        n216 = call "获取最近两组水样测试数据.vi"("error in (no error)"=w416, "table"="pH") -> ("error out"=w420:errorcluster, "存储变量"=w419:T14)  [unwired: 8 in]
                        n217 = call "集成干预测试数据存储.vi"("error in (no error)"=w420, "存储变量"=w419) -> ("error out"=w417:errorcluster)  [unwired: 9 in]
                      }
                    }
                    n218 = case shown="真" w382 {
                      tunnel: [_ w412] -> w381
                      tunnel: w384 -> [_ w411]
                      frame False {
                      }
                      frame True {
                        n219 = call "获取最近两组水样测试数据.vi"("error in (no error)"=w411, "table"="DO") -> ("error out"=w415:errorcluster, "存储变量"=w414:T14)  [unwired: 8 in]
                        n220 = call "集成干预测试数据存储.vi"("error in (no error)"=w415, "存储变量"=w414) -> ("error out"=w412:errorcluster)  [unwired: 9 in]
                      }
                    }
                    n221 = case shown="真" w379 {
                      tunnel: [_ w407] -> w375
                      tunnel: w381 -> [_ w406]
                      frame False {
                      }
                      frame True {
                        n222 = call "获取最近两组水样测试数据.vi"("error in (no error)"=w406, "table"="比电导率") -> ("error out"=w410:errorcluster, "存储变量"=w409:T14)  [unwired: 8 in]
                        n223 = call "集成干预测试数据存储.vi"("error in (no error)"=w410, "存储变量"=w409) -> ("error out"=w407:errorcluster)  [unwired: 9 in]
                      }
                    }
                    n224 = case shown="真" w374 {
                      tunnel: [_ w402] -> w373
                      tunnel: w375 -> [_ w401]
                      frame False {
                      }
                      frame True {
                        n225 = call "获取最近两组水样测试数据.vi"("error in (no error)"=w401, "table"="浊度") -> ("error out"=w405:errorcluster, "存储变量"=w404:T14)  [unwired: 8 in]
                        n226 = call "集成干预测试数据存储.vi"("error in (no error)"=w405, "存储变量"=w404) -> ("error out"=w402:errorcluster)  [unwired: 9 in]
                      }
                    }
                    n227 = case shown="真" w372 {
                      tunnel: [_ w397] -> w371
                      tunnel: w373 -> [_ w396]
                      frame False {
                      }
                      frame True {
                        n228 = call "获取最近两组水样测试数据.vi"("error in (no error)"=w396, "table"="叶绿素") -> ("error out"=w400:errorcluster, "存储变量"=w399:T14)  [unwired: 8 in]
                        n229 = call "集成干预测试数据存储.vi"("error in (no error)"=w400, "存储变量"=w399) -> ("error out"=w397:errorcluster)  [unwired: 9 in]
                      }
                    }
                    n230 = case shown="真" w370 {
                      tunnel: [_ w392] -> _
                      tunnel: w371 -> [_ w391]
                      frame False {
                      }
                      frame True {
                        n231 = call "获取最近两组水样测试数据.vi"("error in (no error)"=w391, "table"="藻密度") -> ("error out"=w395:errorcluster, "存储变量"=w394:T14)  [unwired: 8 in]
                        n232 = call "集成干预测试数据存储.vi"("error in (no error)"=w395, "存储变量"=w394) -> ("error out"=w392:errorcluster)  [unwired: 9 in]
                      }
                    }
                  }
                }
              }
            }
          }
        }
        n233 = global read "采配水全局变量.vi" "状态"() -> (w271:T9)
        n234 = Unbundle By Name(w271) -> ("R0"=w270:i16)
        n235 = Equal To 0?(x=w270) -> (x = 0?=w269:bool)
        n236 = Select(t=enum16{"初始化", "采配水启动", "仪器操作", "反冲洗", "结束"}."结束" ("枚举"), s=w269, f=enum16{"初始化", "采配水启动", "仪器操作", "反冲洗", "结束"}."反冲洗" ("枚举")) -> (s? t:f=w266:enum16{"初始化", "采配水启动", "仪器操作", "反冲洗", "结束"})
      }
      frame "结束" {
        n237 = Release Queue(queue=w442) -> ()  [unwired: 2 in, 3 out]
        n238 = Unbundle By Name(w439) -> ("测试模式"=w440:enum16{"正常测试", "集成干预"})
        n239 = Cancel Notification(0:w443) -> (8:w444:refnum<notifier>)  [unwired: 1 in, 2 out]
        n240 = Release Notifier(notifier=w444) -> ()  [unwired: 2 in, 3 out]
        n241 = case shown="\"集成干预\"" w440 {
          tunnel: w438 -> [_ w447]
          frame "正常测试", Default {
          }
          frame "集成干预" {
            n242 = global write "系统设置全局变量.vi" "运行模式"(w447) -> ()
          }
        }
      }
    }
    n243 = Format Into String(format string="%s,当前运行时间%d秒" ("格式字符串"), w15, w11) -> (resulting string=w16:string)  [unwired: 2 in, 1 out]
    n244 = global write "采配水全局变量.vi" "运行状态显示"(w16) -> ()
  }
